vi "Read SSH.vi"(8 "Error In":errorcluster, 11 "Agent In":refnum<class "Agent.lvclass">) -> (0 "Error Out":errorcluster, 2 "SSH":refnum<class "SSH.lvclass">, 3 "Agent Out":refnum<class "Agent.lvclass">)   [LabVIEW 2018, in "Toolkit.lvlib" / "Agent.lvclass"]
uses:
  Agent.lvclass
  SSH/SSH.lvclass
  Agent.lvclass/Agent.ctl
  Session/Session.lvclass/Session.ctl
  Session/Session.lvclass
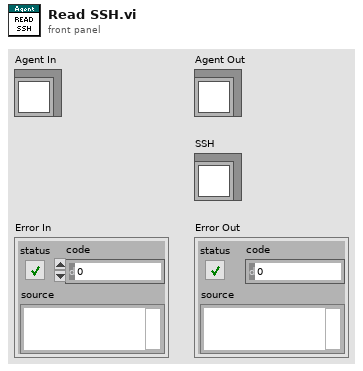
[diagram p1: front panel]
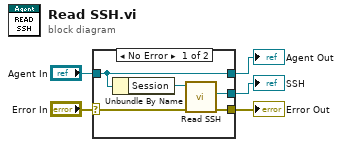
[diagram p0: block diagram]
diagram:
  n1 = case shown="No Error" "Error In" {
    selector: "Error In" -> [w8 w11]
    tunnel: "Agent In" -> [w10 w12]
    tunnel: [w10 w12] -> w1
    tunnel: [w6 w11] -> w4
    tunnel: [w7 _] -> w3
    frame No Error {
      n2 = Unbundle By Name(w10) -> ("Session"=w9:refnum<class "Session.lvclass">)
      n3 = call "Read SSH.vi"("Error In"=w8, "Session In"=w9) -> ("Erorr Out"=w6:errorcluster, "SSH"=w7:refnum<class "SSH.lvclass">)  [unwired: 7 in, 1 out]
    }
    frame Error {
    }
  }
  "Error Out" <- w4
  "SSH" <- w3
  "Agent Out" <- w1
